vi "Win32 Open File.vi"(8 "error in (no error)":errorcluster, 9 "desired access (read & write)":u32(ring)=3221225472 items=["read"=2147483648, "write"=1073741824, "read & write"=3221225472, "execute"=536870912, "all"=268435456], 10 "creation mode (open)":T1(ring)=enum."OPEN_EXISTING (open)", 11 "file path":path) -> (0 "error out":errorcluster, 2 "Windows file handle out":u32, 3 "LabVIEW file refnum out":refnum<file>)   [LabVIEW 2013]
doc: "This VI opens or creates a file using the Win32 CreateFile function in a way that disables the Windows file cache for the specified file, leading to greater performance for sequential reads and writes. This VI provides a reference to the file opened as a <b>LabVIEW file refnum</b>, allowing you to interact with the file using the standard LabVIEW File I/O functions, and also provides a reference to the file as a <b>Windows file handle</b>, for use with the associated Win32 File I/O VIs.\n\n<b>Note! With Windows file caching disabled by this VI, all reads and writes to this file must be made in increments of the sector size of the disk (typically 512 bytes).</b>\n\n<b>Details</b>\nThis VI disables Windows file caching by setting the FILE_FLAG_NO_BUFFERING flag when opening or creating the file. After opening the file in this special fashion, it calls into a LabVIEW entry point to convert the Windows file handle to a LabVIEW file refnum, allowing for use of all of the LabVIEW file I/O primitives. This should work well for most applications. \n\nHowever, if your read performance is not matching the physical limits of your hard drive or RAID array system (run the Win32 Read From File Speed Test Reallocated Array), you may need to make use of the special Win32 Read VIs distributed along with this VI. The special Win32 Read VIs read data into a pre-allocated buffer, avoiding the allocation of an array each time data is read.\n\nIt is required that the memory for the data be aligned on certain memory boundaries, depending on the requirements of the hard disk controller or RAID controller in your system. Most controllers have memory alignment requirements of 1, 2, 4, or 8 bytes. It is not possible in LabVIEW to specify memory alignment for arrays, although most LabVIEW arrays are aligned on 8-byte boundaries. If these Win32 File I/O VIs produce unexpected or undefined errors, memory alignment and unbuffered file I/O may be an issue on your system and you may need to use a different hard disk controller or RAID controller."
uses:
  kernel32.dll
panel:
  in  "File Refnum":refnum<file>
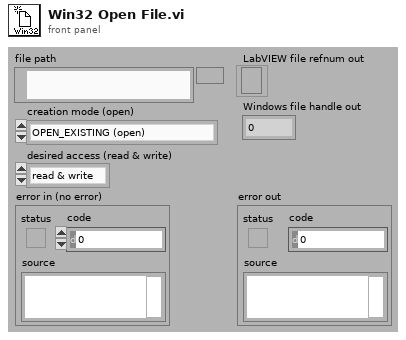
[diagram p1: front panel]
types:
  T1 = enum32{"CREATE_NEW (create)", "CREATE_ALWAYS (replace or create)", "OPEN_EXISTING (open)", "OPEN_ALWAYS (open or create)", "TRUNCATE_EXISTING (replace)"}
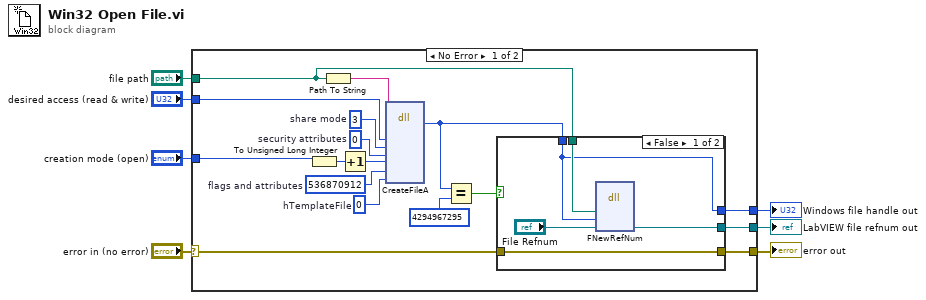
[diagram p0: block diagram]
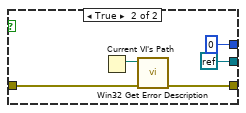
[diagram p2: hidden frame]
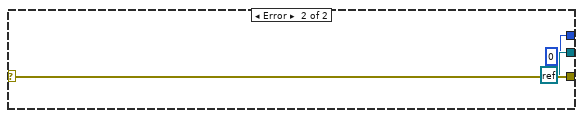
[diagram p3: hidden frame]
diagram:
  n1 = case shown="No Error" "error in (no error)" {
    selector: "error in (no error)" -> [w23 w37]
    tunnel: [w22 w37] -> w6
    tunnel: "file path" -> [w13 _]
    tunnel: "desired access (read & write)" -> [w12 _]
    tunnel: "creation mode (open)" -> [w11 _]
    tunnel: [w10 refnum<k0> refnum] -> w3
    tunnel: [w9 u32 0 ("FileDescriptor")] -> w2
    frame No Error {
      w20 = u32 0  # security attributes
      w19 = u32 0  # hTemplateFile
      w17 = u32 536870912  # flags and attributes
      w15 = u32 3  # share mode
      n2 = To Unsigned Long Integer(number=w11) -> (unsigned 32bit integer=w18:u32)
      n3 = Path To String(path=w13) -> (string=w8:string)
      n4 = Increment(x=w18) -> (x+1=w16:u32)
      n5 = dll-call lib="kernel32.dll" fn="CreateFileA"("lpFileName"=w8, "dwDesiredAccess"=w12, "dwShareMode"=w15, "lpSecurityAttributes"=w20, "dwCreationDisposition"=w16, "dwFlagsAndAttributes"=w17, "hTemplateFile"=w19) -> (w14:u32)  [unwired: 10 in, 2 out]
      n6 = Equal?(x=w14, y=u32 4294967295) -> (x = y?=w21:bool)
      n7 = case shown="False" w21 {
        tunnel: w23 -> [w29 w31]
        tunnel: [w29 w30] -> w22
        tunnel: w13 -> [w27 _]
        tunnel: w14 -> [w25 _]
        tunnel: [w26 refnum<k0> refnum] -> w10
        tunnel: [w25 u32 0 ("FileDescriptor")] -> w9
        frame False {
          n8 = dll-call lib="LabVIEW" fn="FNewRefNum"("file path"=w27, "FileDescriptor"=w25, "File Refnum"="File Refnum") -> ("File Refnum"=w26:refnum<file>)  [unwired: 6 in, 2 out]
        }
        frame True {
          n9 = Current VI's Path() -> (path=w32:path)
          n10 = call "Win32 Get Error Description.vi"("error in (no error)"=w31, "current VI's path"=w32) -> ("error out"=w30:errorcluster)  [unwired: 7 in, 2 out]
        }
      }
    }
    frame Error {
    }
  }
  "error out" <- w6
  "LabVIEW file refnum out" <- w3
  "Windows file handle out" <- w2
